vi "wavelength scan_Rb_v1.0.vi"() -> ()   [LabVIEW 2012]
panel:
  out "Waveform Chart 2":dbl(graph)=0.001003
  in  "onlineTEC_offset":dbl=0.012 format="%.4g"
  out "Lambda Read (nm)":dbl=780.2412915934927 format="%.5f"
  out "Wavelength Lock":bool=TRUE
  out "XY Graph":cluster{"Y":dbl[], "Y":dbl[]}[](graph)
  out "Power (W)":dbl=0.001003 format="%.3p"
  out "OphirPM":T1={"Ophir-Ref"=refnum, "Ophir-Device"=1000, "Ophir-Channel"=0}
  out "Waveform Chart":dbl(graph)=780.2412915934927
  in  "Lambda Step (nm)":dbl=5e-05 format="%.5f"
  in  "Lambda Stop (nm)":dbl=780.25 format="%.5f"
  in  "Lambda Start (nm)":dbl=780.23 format="%.5f"
  in  "step_size":dbl=0.0005 format="%#_6p"
  in  "Device In":refnum<visa-resource-name>="TL_Pro800"
  in  "Settings":T2={"Module"=enum."On Line TEC", "OnLineTEC"=15.3, "OnLineLD"=0.1} {"OnLineLD" min=0.0 max=0.175 step=0.001 format="%.3p"; "OnLineTEC" min=0.0 max=30.0 step=0.1 format="%.3g"}
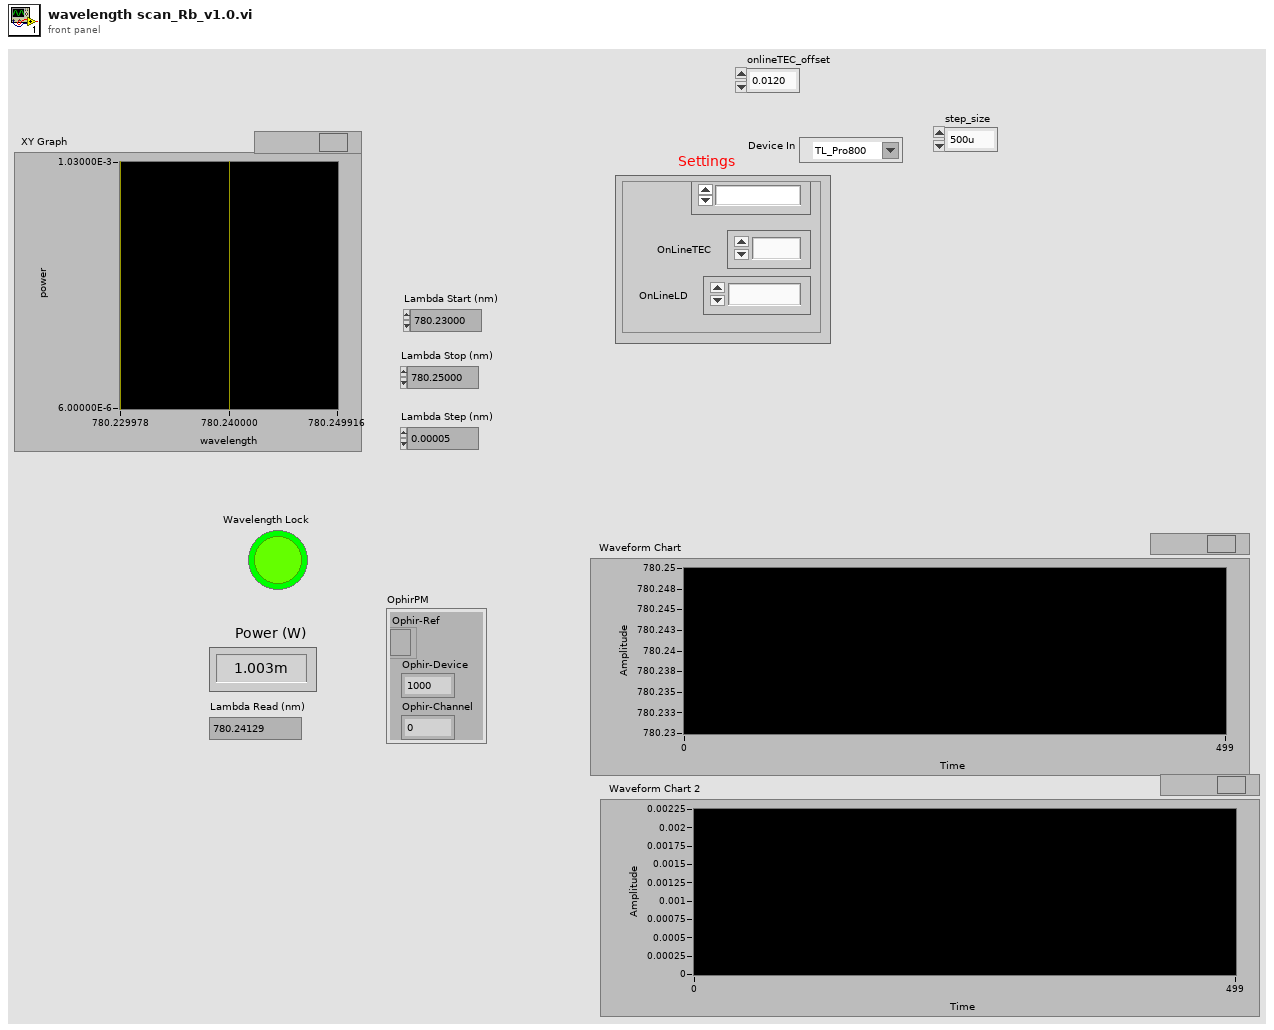
[diagram p1: front panel]
types:
  T1 = cluster{"Ophir-Ref":refnum<k7>, "Ophir-Device":i32, "Ophir-Channel":i32}
  T2 = cluster{"Module":enum16{"On Line TEC", "On Line LD"}, "OnLineTEC":dbl, "OnLineLD":dbl}
  T3 = enum16{"Open_TL", "Close_TL", "Verify_ID", "TEC_Sensor", "SET", "READ", "ON", "OFF", "Read_Status"}
  T4 = enum16{"On Line TEC", "On Line LD", "Off Line TEC", "Off Line LD", "Etalon TEC", "TSOA TEC"}
  T5 = cluster{"OnLineTEC":dbl, "OnLineLD":dbl, "OffLineTEC":dbl, "OffLineLD":dbl, "EtalonTEC":dbl, "TSOA-TEC":dbl, "Pro800":bool, "OnLine TEC":bool, "OnLine LD":bool, "nothing":bool, "nothing":bool, "nothing":bool, "nothing":bool}
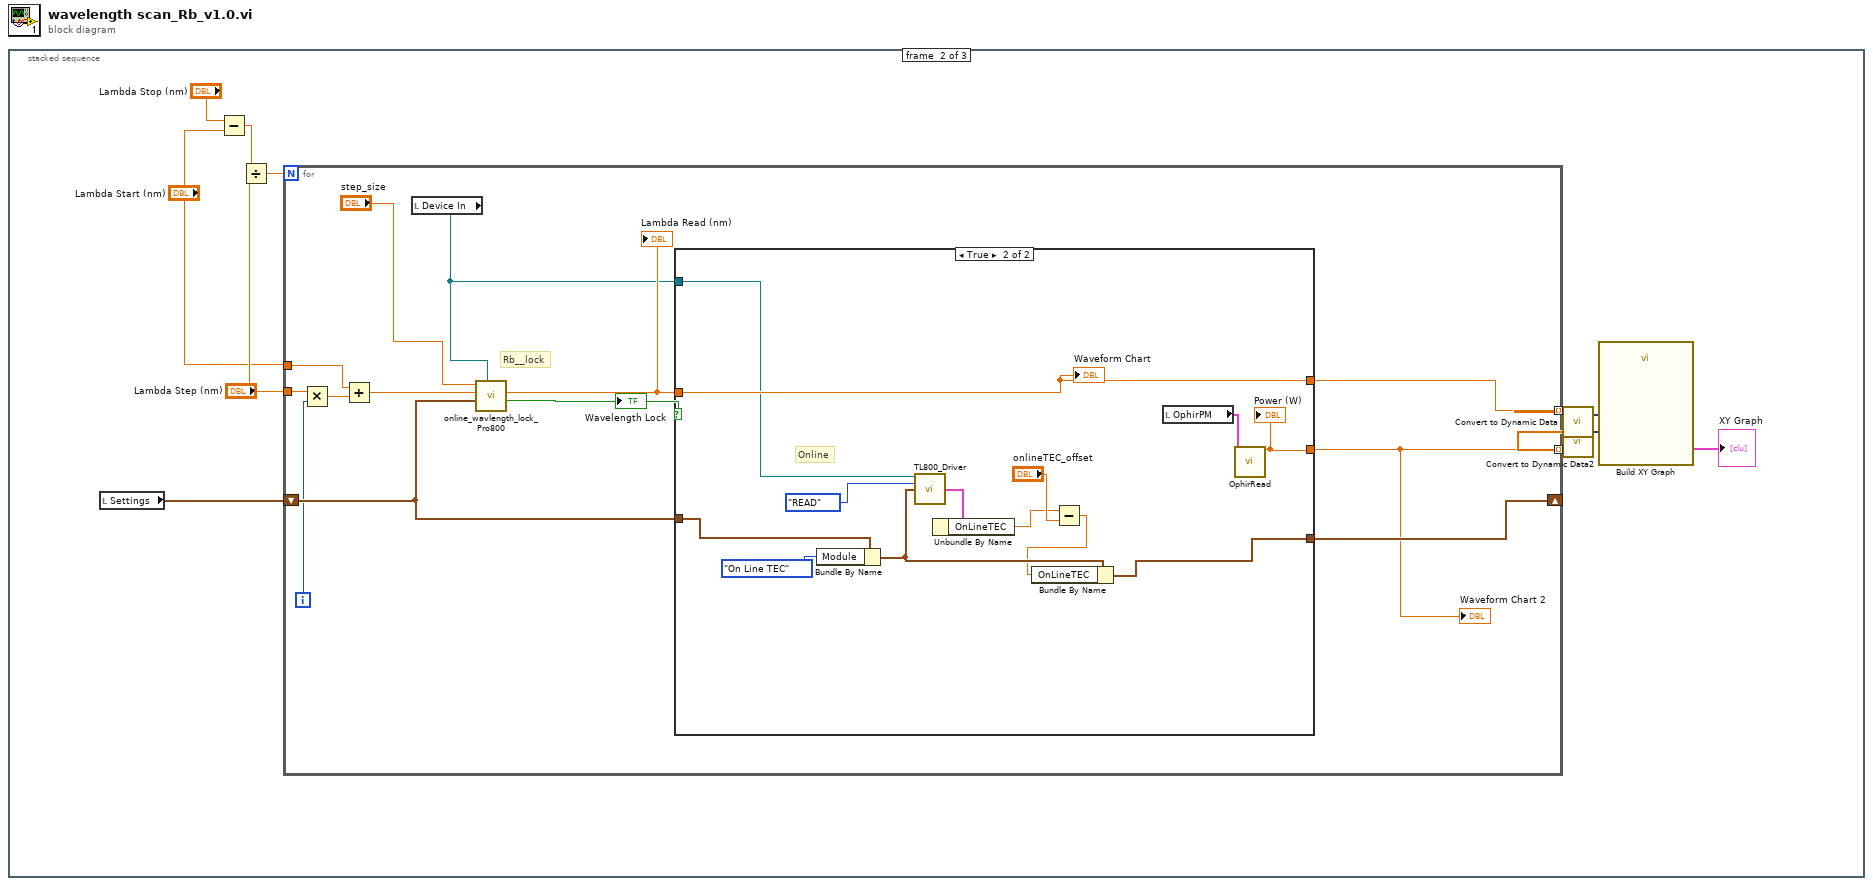
[diagram p0: block diagram]
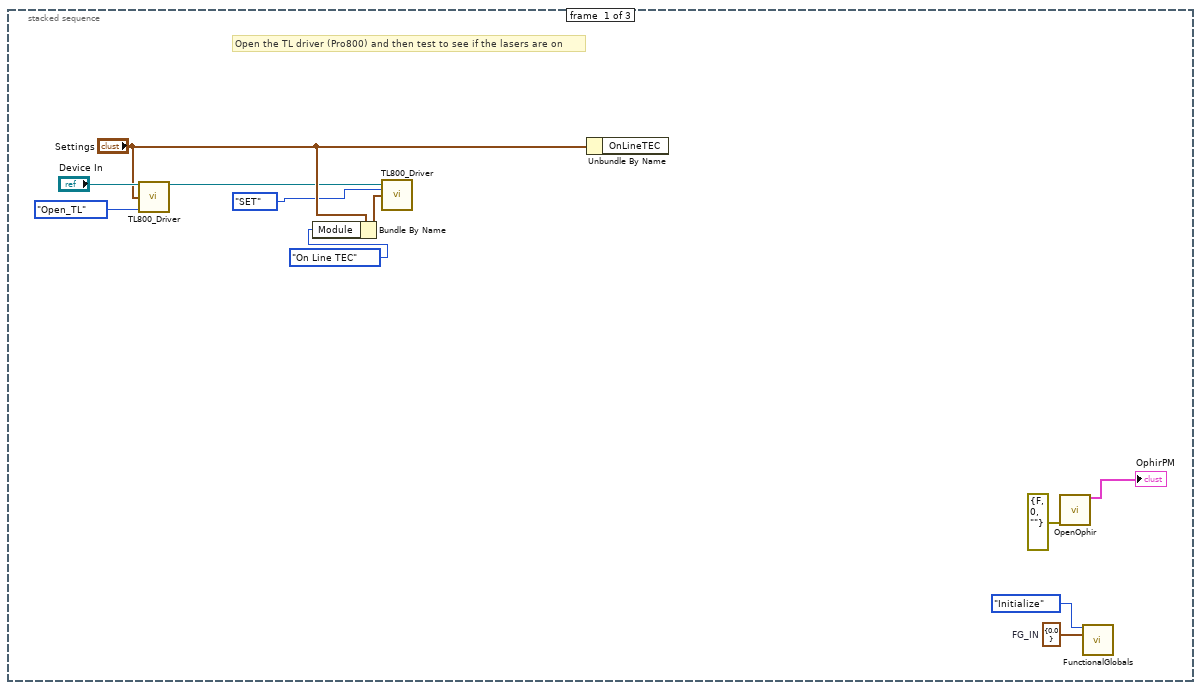
[diagram p2: hidden frame]
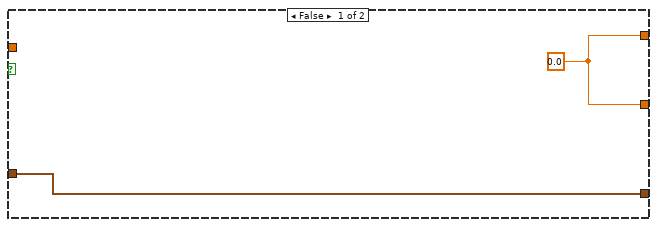
[diagram p3: hidden frame]
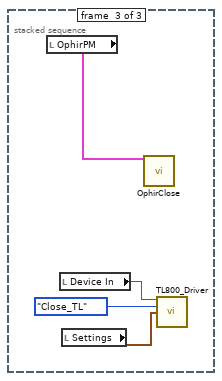
[diagram p4: hidden frame]
diagram:
  n1 = stacked-sequence {
    frame #0 {
      w8 = cluster{"PowerIn":dbl} {"PowerIn"=0.0}  # FG_IN
      # "Open the TL driver (Pro800) and then test to see if the lasers are on"
      n2 = call "TL800_Driver.vi"("Device In"="Device In", "Commands"=T3."Open_TL", "Settings"="Settings") -> ("Device Out"=w3:refnum<visa-resource-name>)  [unwired: 9 in, 3 out]
      n3 = Bundle By Name(cluster="Settings", "Module"=T4."On Line TEC") -> (w6:T2)
      n4 = call "TL800_Driver.vi"("Device In"=w3, "Commands"=T3."SET", "Settings"=w6) -> ()  [unwired: 9 in, 4 out]
      n5 = Unbundle By Name("Settings") -> ()  [unwired: 1 out]
      n6 = call "OpenOphir.vi"("error in (no error)"=errorcluster {"status"=FALSE, "code"=0, "source"=""}) -> ("OphirPM"=→"OphirPM":T1)  [unwired: 13 in, 1 out]
      n7 = call "FunctionalGlobals.vi"("FG_Control"=enum16{"Initialize", "PowerRead", "PowerWrite"}."Initialize", "FG_IN"=w8) -> ()  [unwired: 13 in, 1 out]
    }
    frame #1 {
      n8 = local read "Settings"() -> (w13:T2)
      n9 = Subtract(x="Lambda Stop (nm)", y="Lambda Start (nm)") -> (x-y=w22:dbl)
      n10 = Divide(x=w22, y="Lambda Step (nm)") -> (x/y=w12:dbl)
      n11 = for {
        N: w12 -> [_]
        tunnel: "Lambda Step (nm)" -> [w35]
        tunnel: "Lambda Start (nm)" -> [w34]
        tunnel: [w24] -> w17 mode=indexing
        tunnel: [w23] -> w15 mode=indexing
        shift-right: [w28] -> _
        shift-left: w13 -> [w26]
        i -> [w25]
        # "Rb__lock"
        n12 = Multiply(x=w35, y=w25) -> (x*y=w33:dbl)
        n13 = Add(x=w34, y=w33) -> (x+y=w32:dbl)
        n14 = local read "Device In"() -> (w27:refnum<visa-resource-name>)
        n15 = call "online_wavlength_lock_Pro800.vi"("Device"=w27, "Settings In"=w26, "Lambda On Set (nm)"=w32, "step_size"="step_size") -> ("Wavelength Lock Online"=w30:bool, "Lambda On Read (nm)"=w29:dbl)  [unwired: 3 in]
        "Wavelength Lock" <- w30
        "Lambda Read (nm)" <- w29
        n16 = case shown="True" w30 {
          tunnel: w29 -> [_ w49]
          tunnel: [w37 w49] -> w24
          tunnel: [w37 w48] -> w23
          tunnel: [w36 w45] -> w28
          tunnel: w27 -> [_ w47]
          tunnel: w26 -> [w36 w46]
          frame False {
            w37 = 0.0
          }
          frame True {
            # "Online"
            n17 = Bundle By Name(cluster=w46, "Module"=T4."On Line TEC") -> (w42:T2)
            n18 = call "TL800_Driver.vi"("Device In"=w47, "Commands"=T3."READ", "Settings"=w42) -> ("Readings"=w43:T5)  [unwired: 9 in, 3 out]
            n19 = Unbundle By Name(w43) -> ("OnLineTEC"=w40:dbl)
            n20 = Subtract(x=w40, y="onlineTEC_offset") -> (x-y=w39:dbl)
            n21 = Bundle By Name(cluster=w42, "OnLineTEC"=w39) -> (w45:T2)
            n22 = local read "OphirPM"() -> (w50:T1)
            n23 = call "OphirRead.vi"("OphirPM"=w50) -> ("Power (W)"=w48:dbl)  [unwired: 12 in, 2 out]
            "Power (W)" <- w48
            "Waveform Chart" <- w49
          }
        }
        "Waveform Chart 2" <- w23
      }
      n24 = call "Convert to Dynamic Data"("Array"=w17) -> ("Dynamic Data Type"=w16:dynamicdata)  [unwired: 3 in]
      n25 = call "Convert to Dynamic Data2"("Array"=w15) -> ("Dynamic Data Type"=w14:dynamicdata)  [unwired: 3 in]
      n26 = call "Build XY Graph"("Y Input"=w14, "X Input"=w16) -> ("XY Graph"=→"XY Graph":cluster{"Y":dbl[], "Y":dbl[]}[])  [unwired: 3 in, 6 out]
    }
    frame #2 {
      n27 = local read "OphirPM"() -> (w54:T1)
      n28 = local read "Device In"() -> (w52:refnum<visa-resource-name>)
      n29 = local read "Settings"() -> (w53:T2)
      n30 = call "OphirClose.vi"("OphirPM"=w54) -> ()  [unwired: 18 in, 1 out]
      n31 = call "TL800_Driver.vi"("Device In"=w52, "Commands"=T3."Close_TL", "Settings"=w53) -> ()  [unwired: 9 in, 4 out]
    }
  }
